vi "AutoCreateNewTableForPaper1_TreePage(SubVI).vi"(10 "NameOfTable":string, 11 "connection reference":T1) -> (3 "Refnum out":T1)   [LabVIEW 2013]
uses:
  <vilib>/addons/database/Auxilliary.llb/DB Tools Column Info.ctl
  <vilib>/addons/database/Auxilliary.llb/DB Tools DataTypes.ctl
  <vilib>/addons/database/Connection.llb/Conn ObjectReference.ctl
  <vilib>/addons/database/NI_Database_API.lvlib
panel:
  in  "Paper1":T2[](array[typedef])=[{"column name"="Questions_Ordered", "data type"=enum."String", "size"=50, "allow null?"=TRUE}, {"column name"="A", "data type"=enum."String", "size"=50, "allow null?"=TRUE}, {"column name"="B", "data type"=enum."String", "size"=50, "allow null?"=TRUE}, {"column name"="C", "data type"=enum."String", "size"=0, "allow null?"=TRUE}, {"column name"="D", "data type"=enum."String", "size"=0, "allow null?"=TRUE}, {"column name"="Question", "data type"=enum."String", "size"=0, "allow null?"=TRUE}, {"column name"="Why", "data type"=enum."String", "size"=0, "allow null?"=TRUE}, {"column name"="Answer", "data type"=enum."String", "size"=0, "allow null?"=TRUE}, {"column name"="Choice", "data type"=enum."String", "size"=0, "allow null?"=TRUE}, {"column name"="Score", "data type"=enum."String", "size"=0, "allow null?"=TRUE}, {"column name"="CurrentQuestionName", "data type"=enum."String", "size"=0, "allow null?"=TRUE}]
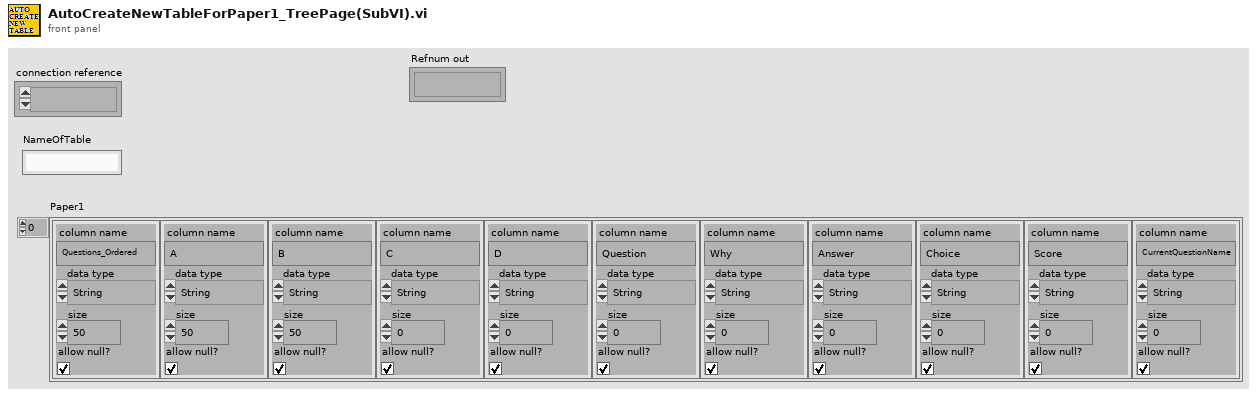
[diagram p1: front panel]
types:
  T1 = typedef "NI_Database_API.lvlib/Conn ObjectReference.ctl" = refnum<k1>
  T2 = typedef "NI_Database_API.lvlib/DB Tools Column Info.ctl" = cluster{"column name":string, "data type":T3, "size":i32, "allow null?":bool}
  T3 = typedef "NI_Database_API.lvlib/DB Tools DataTypes.ctl" = enum16{"String", "Long (I32)", "Single (SGL)", "Double (DBL)", "Date/Time", "Binary"}
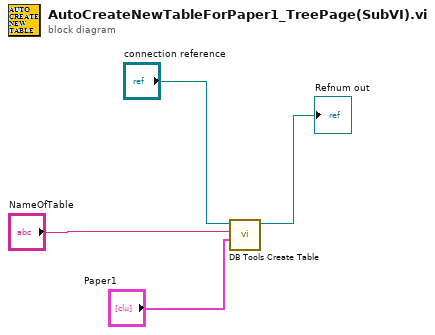
[diagram p0: block diagram]
diagram:
  n1 = call <vilib>:"DB Tools Create Table.vi"("column information"="Paper1", "table"="NameOfTable", "connection reference"="connection reference") -> ("connection reference out"=→"Refnum out":T1)  [unwired: 5 in, 1 out]
